vi "Initialize Categories.vi"(8 "error in (no error)":errorcluster, 11 "Cats XML":path=path "C:/Users/frmausse/Desktop/Summer Projects/VIStore (Actor)/Source/StoreCats.xml") -> (0 "error out":errorcluster, 3 "All Categories":refnum<class "Category.lvclass">[](array[class]))   [LabVIEW 2015, in "VI App Store.lvlib" / "VIStore.lvclass"]
uses:
  VIStore.lvclass
  Classes/Category/Category.lvclass
  Classes/Home/Home.lvclass
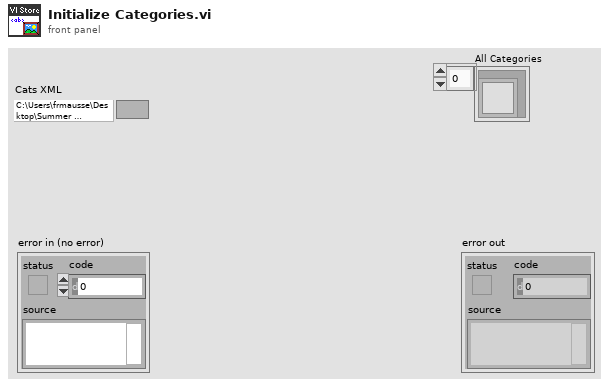
[diagram p1: front panel]
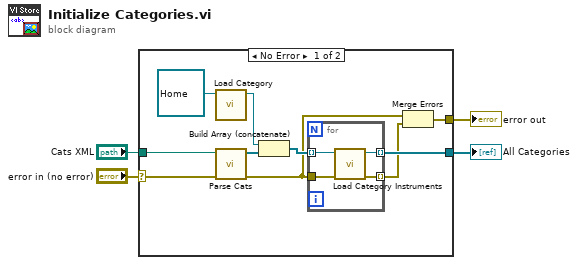
[diagram p0: block diagram]
diagram:
  n1 = case shown="No Error" "error in (no error)" {
    selector: "error in (no error)" -> [w13 w19]
    tunnel: [w8 w19] -> w3
    tunnel: "Cats XML" -> [w7 _]
    tunnel: [w11 _] -> w1
    frame No Error {
      n2 = call-dynamic "Load Category.vi"("Home in"=refnum<class "Home.lvclass"> refnum ("Home.lvclass")) -> ("Home out"=w5:refnum<class "Home.lvclass">)  [unwired: 9 in, 1 out]
      n3 = call "Parse Cats.vi"("error in (no error)"=w13, "path to XML document"=w7) -> ("error out"=w10:errorcluster, "Categories"=w14:refnum<class "Category.lvclass">[])  [unwired: 8 in]
      n4 = Build Array (concatenate)(w5, w14) -> (w12:refnum<class "Category.lvclass">[])
      n5 = for {
        tunnel: w12 -> [w18] mode=indexing
        tunnel: [w17] -> w11 mode=indexing
        tunnel: w10 -> [w16]
        tunnel: [w15] -> w9 mode=indexing
        n6 = call-dynamic "Load Category Instruments.vi"("error in (no error)"=w16, "Category in"=w18) -> ("error out"=w15:errorcluster, "Category out"=w17:refnum<class "Category.lvclass">)  [unwired: 8 in]
      }
      n7 = Merge Errors(w10, w9) -> (w8:errorcluster)
    }
    frame Error {
    }
  }
  "error out" <- w3
  "All Categories" <- w1
